vi "LINC Register Reference.vi"(4 "alternate data names (empty)":string[](array[string]), 5 "ID":i32=-1, 6 "alternate packet names (empty)":string[](array[string]), 7 "single packet (F)":bool, 8 "error in (no error)":errorcluster, 9 "type (CMD)":enum16{"CMD", "TLM", "CMD_HDR", "TLM_HDR"}(ring), 10 "controls":refnum<vi>[](array[refnum]), 11 "LINC session":refnum<class "LINC.lvclass">) -> (0 "error out":errorcluster, 3 "dup LINC session":refnum<class "LINC.lvclass">)   [LabVIEW 2018, in "STEPkgDriver_LINC.lvlib" / "LINC.lvclass"]
uses:
  LINC.lvclass
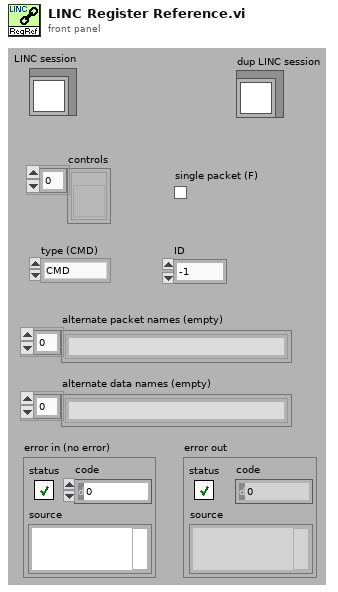
[diagram p1: front panel]
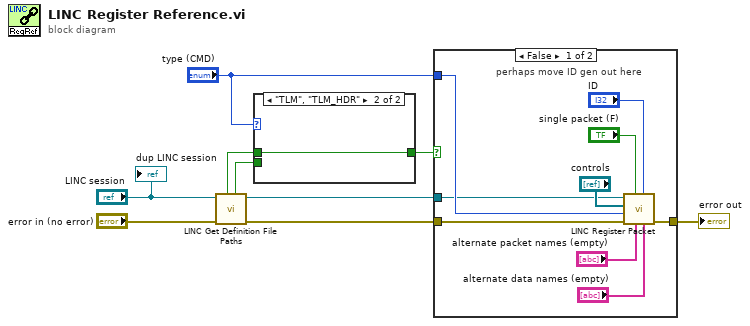
[diagram p0: block diagram]
diagram:
  n1 = call "LINC Get Definition File Paths.vi"("error in (no error)"="error in (no error)", "LINC session"="LINC session") -> ("error out"=w6:errorcluster, "dup LINC session"=w4:refnum<class "LINC.lvclass">, "CMD definition exists"=w1:bool, "TLM definition exists"=w2:bool)  [unwired: 4 in, 2 out]
  n2 = case shown="\"TLM\", \"TLM_HDR\"" "type (CMD)" {
    tunnel: w2 -> [_ w11]
    tunnel: w1 -> [w10 _]
    tunnel: [w10 w11] -> w5
    frame "CMD", "CMD_HDR" {
    }
    frame "TLM", "TLM_HDR" {
    }
  }
  n3 = case shown="False" w5 {
    tunnel: "type (CMD)" -> [w15 _]
    tunnel: [w14 w21] -> w8
    tunnel: w6 -> [w13 w21]
    tunnel: w4 -> [w12 _]
    frame False {
      # "perhaps move ID gen out here"
      n4 = call "LINC Register Packet.vi"("alternate data names (empty)"="alternate data names (empty)", "ID"="ID", "alternate packet names (empty)"="alternate packet names (empty)", "single packet (F)"="single packet (F)", "error in (no error)"=w13, "type (CMD)"=w15, "controls"="controls", "LINC session"=w12) -> ("error out"=w14:errorcluster)  [unwired: 2 in, 1 out]
    }
    frame True {
    }
  }
  "error out" <- w8
  "dup LINC session" <- "LINC session"
